vi "Parse params.vi"(9 "error in (no error)":errorcluster, 10 "params":variant) -> (1 "error out":errorcluster, 2 "data":dbl[](array[numeric]))   [LabVIEW 2016, in "JSON-RPC.lvclass"]
uses:
  JSON-RPC.lvclass
  <vilib>/Utility/Data Type/NI_Data Type.lvlib
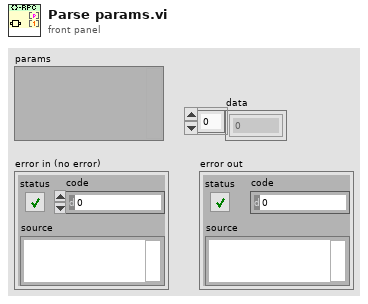
[diagram p1: front panel]
types:
  T1 = typedef "NI_Data Type.lvlib/Data Type.ctl" = enum8{"Invalid Type", "Void", "I8", "I16", "I32", "I64", "U8", "U16", "U32", "U64", "Single Float", "Double Float", "Extended Float", "Single Complex", "Double Complex", "Extended Complex", "Enum U8", "Enum U16", "Enum U32", "Enum U64", "Single Float With Unit", "Double Float With Unit", "Extended Float With Unit", "Single Complex with Unit", "Double Complex with Unit", "Extended Complex with Unit", "Boolean", "String", "Path", "Picture", "Tag", "Array", "Cluster", "Variant", "LV Variant", "Waveform", "Timestamp", "Digital Waveform", "Digital Data", "ExpressData", "Refnum", "External Data", "VI", "Poly VI", "LabVIEW Class Instance", "Fixed Point"}
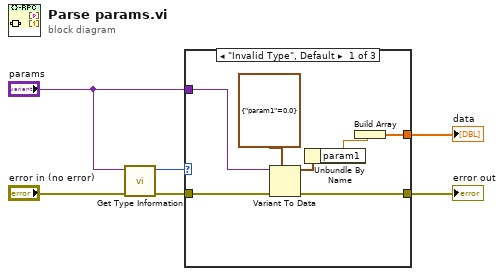
[diagram p0: block diagram]
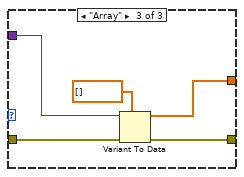
[diagram p3: hidden frame]
diagram:
  n1 = call <vilib>:"Get Type Information.vi"("error in (no error)"="error in (no error)", "Variant"="params") -> ("error out"=w2:errorcluster, "Type"=w4:T1)  [unwired: 5 in, 3 out]
  n2 = case shown="\"Invalid Type\", Default" w4 {
    tunnel: [w12 w14 w19] -> w6
    tunnel: w2 -> [w13 w14 w17]
    tunnel: "params" -> [w11 _ w15]
    tunnel: [w7 _ w16] -> w1
    frame "Invalid Type", Default {
      n3 = Variant To Data(error in=w13, type=cluster{"param1":dbl} {"param1"=0.0}, Variant=w11) -> (data=w9:cluster{"param1":dbl}, error out=w12:errorcluster)
      n4 = Unbundle By Name(w9) -> ("param1"=w8:dbl)
      n5 = Build Array(w8) -> (w7:dbl[])
    }
    frame "Cluster" {
    }
    frame "Array" {
      n6 = Variant To Data(error in=w17, type=dbl[] [] ("data"), Variant=w15) -> (data=w16:dbl[], error out=w19:errorcluster)
    }
  }
  "error out" <- w6
  "data" <- w1
